vi "Sort Mode Coefficients SLM.vi"(7 "coefficient source":string="manual modes") -> (8 "coefficient list":dbl[][](array[numeric]))   [LabVIEW 2014]
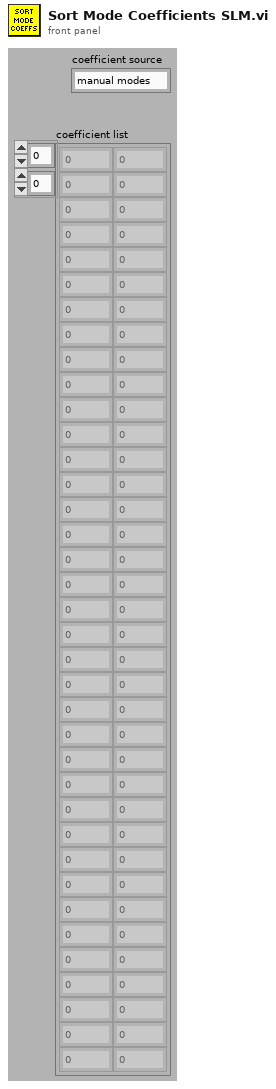
[diagram p1: front panel]
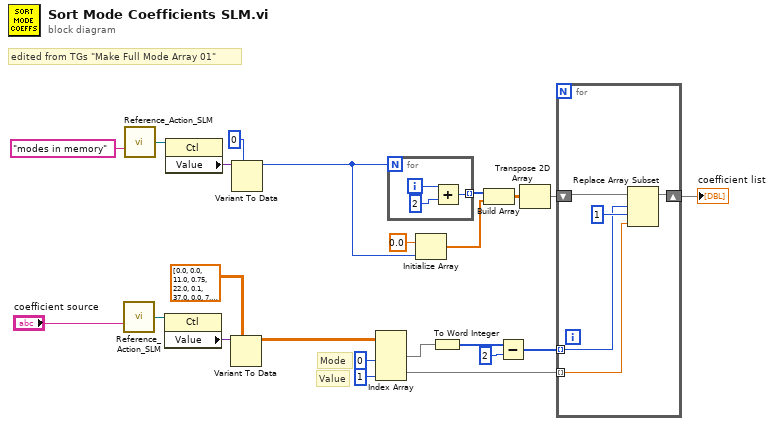
[diagram p0: block diagram]
diagram:
  # "edited from TGs \"Make Full Mode Array 01\""
  # "Value"
  # "Mode"
  n1 = call "Reference_Action_SLM.vi"("Control Name"="coefficient source") -> ("Ref OUT"=w5:refnum<vi>)  [unwired: 12 in, 2 out]
  n2 = call "Reference_Action_SLM.vi"("Control Name"="modes in memory") -> ("Ref OUT"=w9:refnum<vi>)  [unwired: 12 in, 2 out]
  n3 = property class="Ctl"(reference=w5) -> ("Value"=w4:variant)  [unwired: 1 in, 2 out]
  n4 = property class="Ctl"(reference=w9) -> ("Value"=w8:variant)  [unwired: 1 in, 2 out]
  n5 = Variant To Data(type=dbl[][] [[0.0, 0.0], [11.0, 0.75], [22.0, 0.1], [37.0, 0.0], [7.0, 0.15], [8.0, 0.1], [5.0, 0.05], [6.0, 0.0], [9.0, 0.0], [10.0, 0.0], [2.0, 0.0], [3.0, -18.3]] ("Mode Coeffs 2"), Variant=w4) -> (data=w2:dbl[][])  [unwired: 1 in, 1 out]
  n6 = Variant To Data(type=0, Variant=w8) -> (data=w6:i32)  [unwired: 1 in, 1 out]
  n7 = Index Array(array=w2, index (col) #1=0 ("disabled index (col)"), index (col) #2=1 ("index (col)")) -> (element #1=w21:dbl[], element #2=w20:dbl[])  [unwired: 2 in]
  n8 = for {
    N: w6 -> [_]
    tunnel: [w24] -> w18 mode=indexing
    i -> [w26]
    n9 = Add(x=w26, y=2) -> (x+y=w24:i32)
  }
  n10 = Initialize Array(0.0 ("element"), w6) -> (w17:dbl[])
  n11 = To Word Integer(number=w21) -> (16bit integer=w13:i16[])
  n12 = Build Array(w18, w17) -> (w15:dbl[][])
  n13 = Subtract(x=w13, y=2) -> (x-y=w12:i32[])
  n14 = Transpose 2D Array(2D array=w15) -> (transposed array=w14:dbl[][])
  n15 = for {
    tunnel: w12 -> [w27] mode=indexing
    tunnel: w20 -> [w29] mode=indexing
    shift-right: [w28] -> w16
    shift-left: w14 -> [w31]
    n16 = Replace Array Subset(array=w31, new element=w29, index (row)=w27, index (col)=1 ("disabled index (col)")) -> (w28:dbl[][])
  }
  "coefficient list" <- w16
